vi "VICI_6 port 2 pos_switch.vi"(2 "Switch to position (A/B)":enum16{"A", "B"}(ring), 3 "Valve ID":string="1", 4 "Valve COM":refnum<visa-resource-name>="COM8") -> (0 "Current position":string)   [LabVIEW 2023]
panel:
  out "error out":errorcluster
  out "read buffer":string
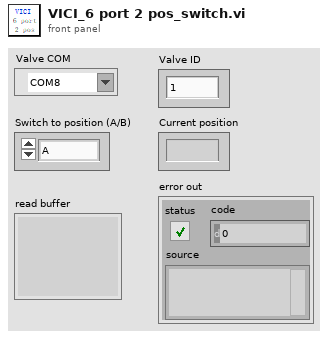
[diagram p1: front panel]
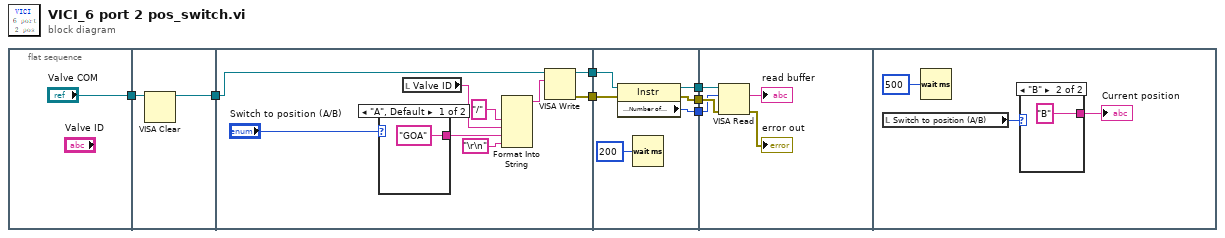
[diagram p0: block diagram]
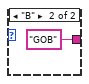
[diagram p2: hidden frame]
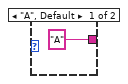
[diagram p3: hidden frame]
diagram:
  n1 = flat-sequence {
    tunnel: ["Valve COM"] -> w2
    tunnel: w2 -> [w10]
    tunnel: [w9] -> w1
    tunnel: [w13] -> w7
    tunnel: [w12] -> w5
    tunnel: w1 -> [w11]
    tunnel: w7 -> [w27]
    tunnel: [w25] -> w6
    tunnel: w5 -> [w26]
    tunnel: [w24] -> w4
    tunnel: [w23] -> w3
    tunnel: w6 -> [w32]
    tunnel: w4 -> [w31]
    tunnel: w3 -> [w30]
    frame #0 {
    }
    frame #1 {
      n2 = VISA Clear(VISA resource name=w10) -> (VISA resource name out=w9:refnum<visa-resource-name>)  [unwired: 1 in, 1 out]
    }
    frame #2 {
      n3 = case shown="\"A\", Default" "Switch to position (A/B)" {
        tunnel: ["GOA" ("input 3") "GOB" ("input 3")] -> w18
        frame "A", Default {
        }
        frame "B" {
        }
      }
      n4 = local read "Valve ID"() -> (w17:string)
      n5 = Format Into String("/", w17, w18, "\r\n") -> (resulting string=w14:string)  [unwired: 3 in, 1 out]
      n6 = VISA Write(VISA resource name=w11, write buffer=w14) -> (VISA resource name out=w13:refnum<visa-resource-name>, error out=w12:errorcluster)  [unwired: 1 in, 1 out]
    }
    frame #3 {
      n7 = property class="Instr"(reference=w27, error in=w26) -> (reference out=w25:refnum<visa-resource-name>, error out=w24:errorcluster, "Serial Settings:Number of Bytes at Serial Port"=w23:u32)
      n8 = Wait (ms)(milliseconds to wait=u32 200) -> ()  [unwired: 1 out]
    }
    frame #4 {
      n9 = VISA Read(VISA resource name=w32, byte count=w30, error in (no error)=w31) -> (read buffer=→"read buffer":string, error out=→"error out":errorcluster)  [unwired: 2 out]
    }
    frame #5 {
      n10 = local read "Switch to position (A/B)"() -> (w35:enum16{"A", "B"})
      n11 = Wait (ms)(milliseconds to wait=u32 500) -> ()  [unwired: 1 out]
      n12 = case shown="\"B\"" w35 {
        tunnel: ["A" ("Current position") "B" ("Current position")] -> w34
        frame "A", Default {
        }
        frame "B" {
        }
      }
      "Current position" <- w34
    }
  }
